vi "Day 22-Calculate Intersection.vi"(10 "Existing in":i64[](array[numeric]), 11 "New in":i64[](array[numeric])) -> (2 "Is there Overlap?":bool, 3 "Intersection out":i64[](array[numeric]))   [LabVIEW 2021]
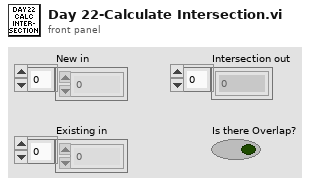
[diagram p1: front panel]
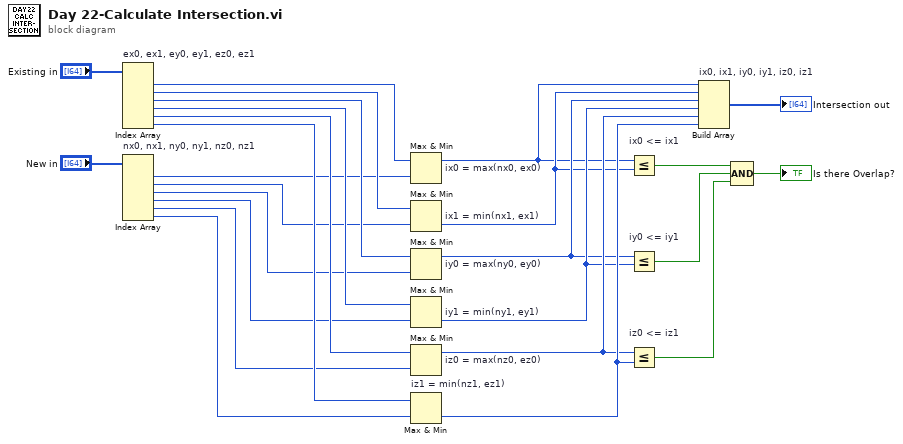
[diagram p0: block diagram]
diagram:
  n1 = Index Array "ex0, ex1, ey0, ey1, ez0, ez1"(array="Existing in") -> (element #1=w2:i64, element #2=w4:i64, element #3=w6:i64, element #4=w8:i64, element #5=w10:i64, element #6=w12:i64)  [unwired: 6 in]
  n2 = Index Array "nx0, nx1, ny0, ny1, nz0, nz1"(array="New in") -> (element #1=w3:i64, element #2=w5:i64, element #3=w7:i64, element #4=w9:i64, element #5=w11:i64, element #6=w13:i64)  [unwired: 6 in]
  n3 = Max & Min "ix0 = max(nx0, ex0)"(x=w2, y=w3) -> (max(x,y)=w19:i64)  [unwired: 1 out]
  n4 = Max & Min "ix1 = min(nx1, ex1)"(x=w4, y=w5) -> (min(x,y)=w20:i64)  [unwired: 1 out]
  n5 = Max & Min "iy0 = max(ny0, ey0)"(x=w6, y=w7) -> (max(x,y)=w21:i64)  [unwired: 1 out]
  n6 = Max & Min "iy1 = min(ny1, ey1)"(x=w8, y=w9) -> (min(x,y)=w22:i64)  [unwired: 1 out]
  n7 = Max & Min "iz0 = max(nz0, ez0)"(x=w10, y=w11) -> (max(x,y)=w24:i64)  [unwired: 1 out]
  n8 = Max & Min "iz1 = min(nz1, ez1)"(x=w12, y=w13) -> (min(x,y)=w25:i64)  [unwired: 1 out]
  n9 = Less Or Equal? "ix0 <= ix1"(x=w19, y=w20) -> (x <= y?=w14:bool)
  n10 = Less Or Equal? "iy0 <= iy1"(x=w21, y=w22) -> (x <= y?=w15:bool)
  n11 = Less Or Equal? "iz0 <= iz1"(x=w24, y=w25) -> (x <= y?=w16:bool)
  n12 = Build Array "ix0, ix1, iy0, iy1, iz0, iz1"(w19, w20, w21, w22, w24, w25) -> (→"Intersection out":i64[])
  n13 = Compound Arithmetic op=AND(w14, w15, w16) -> (→"Is there Overlap?":bool)
